vi "SubVI_Number to Session.vi"(11 "Number":u8) -> (2 "CCD#":string, 3 "Session Out":T1="cam0")   [LabVIEW 2015]
uses:
  <vilib>/userdefined/High Color/IMAQdx.ctl
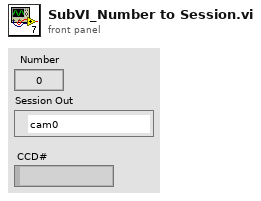
[diagram p1: front panel]
types:
  T1 = typedef "IMAQdx.ctl" = refnum<k21>
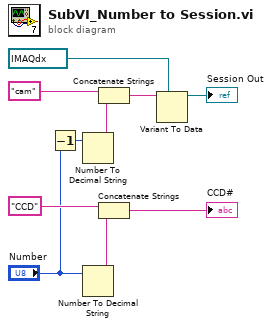
[diagram p0: block diagram]
diagram:
  n1 = Decrement(x="Number") -> (x-1=w1:u8)
  n2 = Number To Decimal String(number=w1) -> (decimal integer string=w3:string)  [unwired: 1 in]
  n3 = Number To Decimal String(number="Number") -> (decimal integer string=w5:string)  [unwired: 1 in]
  n4 = Concatenate Strings("cam", w3) -> (w8:string)
  n5 = Concatenate Strings("CCD", w5) -> (→"CCD#":string)
  n6 = Variant To Data(type=T1 "cam0" ("Session In"), Variant=w8) -> (data=→"Session Out":T1)  [unwired: 1 in, 1 out]
